vi "Am_Init.vi"(0 "COMPORT":refnum<visa-resource-name>="COM4", 1 "file path (dialog if empty)":path=path "C:/TetraLabGUI/Am_Init.py", 11 "error in (no error)":errorcluster, 13 "Open/Close Serial":bool) -> (3 "All Success":bool=TRUE, 4 "comport":refnum<visa-resource-name>="COM4", 15 "error out":errorcluster)   [LabVIEW 2018]
uses:
  <vilib>/Utility/error.llb/whitespace.ctl
  <vilib>/Utility/file.llb/Read Delimited Spreadsheet (string).vi
panel:
  in  "Run TetraSerial(t)":bool=TRUE
  out "size(s)":i32=17
  out "spreadsheet string":string="wr reg 0x02 0x0400;wr reg 0x03 0x0000;wr reg 0x04 1032;wr reg 0x05 4;wr reg 0x06 10;wr reg 0x08 256;wr reg 0x09 51;wr reg 0x0A 4;wr reg 0x0E 8000;wr reg 0x0F 0x5555;wr reg 0x10 0x0055;wr reg 0x11 0xAAAA;wr reg 0x12 0x00AA;wr reg 0x1A 0x0000;wr reg 0x1B 0x0000;wr reg 0x17 0x0300;wr reg 0x18 0x0000\r\n"
  out "Array":string[](array[string])=["wr reg 0x02 0x0400", "wr reg 0x03 0x0000", "wr reg 0x04 1032", "wr reg 0x05 4", "wr reg 0x06 10", "wr reg 0x08 256", "wr reg 0x09 51", "wr reg 0x0A 4", "wr reg 0x0E 8000", "wr reg 0x0F 0x5555", "wr reg 0x10 0x0055", "wr reg 0x11 0xAAAA", "wr reg 0x12 0x00AA", "wr reg 0x1A 0x0000", "wr reg 0x1B 0x0000", "wr reg 0x17 0x0300", "wr reg 0x18 0x0000"]
  out "Numeric":i32=18
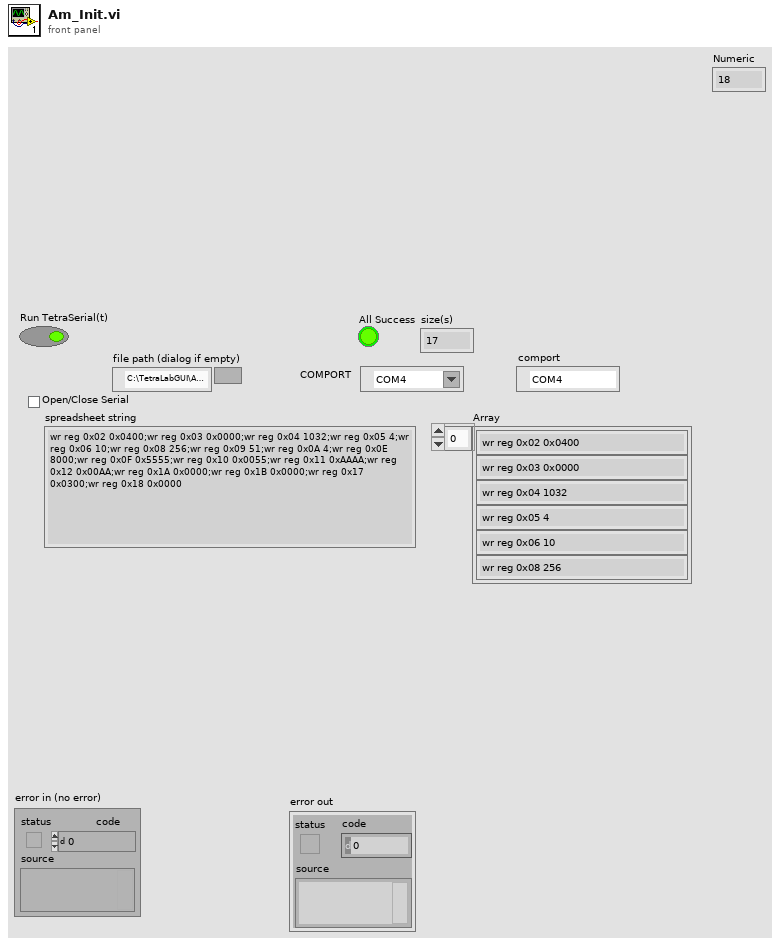
[diagram p1: front panel]
types:
  T1 = typedef "whitespace.ctl" = u16
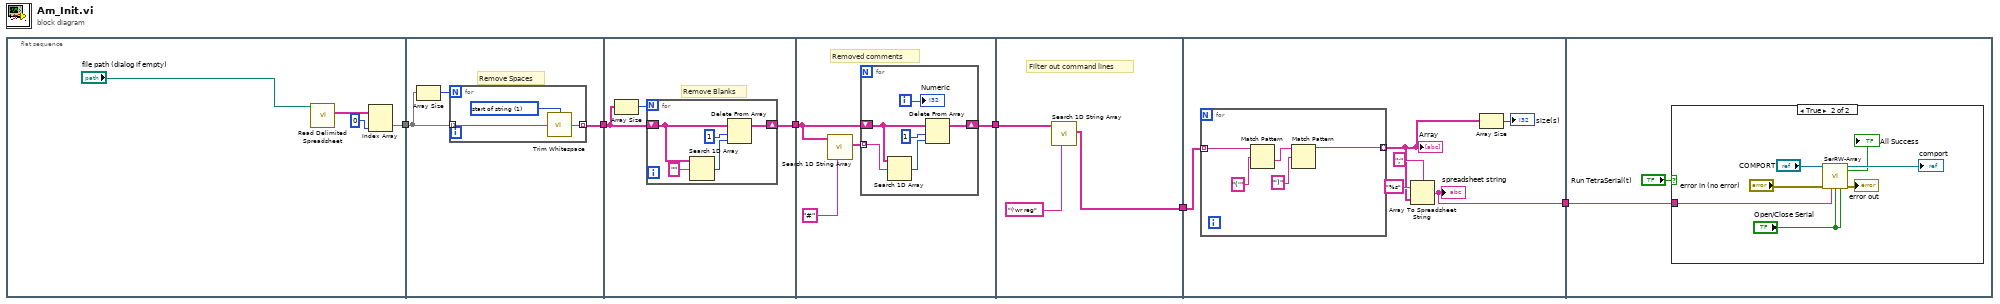
[diagram p0: block diagram]
diagram:
  n1 = flat-sequence {
    tunnel: [w7] -> w6
    tunnel: w6 -> [w12]
    tunnel: [w11] -> w5
    tunnel: w5 -> [w18]
    tunnel: [w17] -> w4
    tunnel: w4 -> [w25]
    tunnel: [w26] -> w3
    tunnel: w3 -> [w36]
    tunnel: [w35] -> w2
    tunnel: w2 -> [w43]
    tunnel: [w40] -> w1
    tunnel: w1 -> [w50]
    frame #0 {
      n2 = call-poly <vilib>:"Read Delimited Spreadsheet.vi"("file path (dialog if empty)"="file path (dialog if empty)") -> ("all rows"=w9:string[][])  [unwired: 9 in, 5 out]
      n3 = Index Array(array=w9, index (col)=0 ("disabled index (col)")) -> (element=w7:string[])  [unwired: 1 in]
    }
    frame #1 {
      # "Remove Spaces"
      n4 = Array Size(array=w12) -> (size(s)=w13:i32)
      n5 = for {
        N: w13 -> [_]
        tunnel: w12 -> [w16] mode=indexing
        tunnel: [w15] -> w11 mode=indexing
        w14 = T1 1 items=["both", "start of string", "end of string"] ("location (both)")
        n6 = call <vilib>:"Trim Whitespace.vi"("string"=w16, "location (both)"=w14) -> ("trimmed string"=w15:string)
      }
    }
    frame #2 {
      # "Remove Blanks"
      n7 = Array Size(array=w18) -> (size(s)=w19:i32)
      n8 = for {
        N: w19 -> [_]
        shift-right: [w21] -> w17
        shift-left: w18 -> [w24]
        n9 = Search 1D Array(1D array=w24, element="") -> (index of element=w23:i32)  [unwired: 1 in]
        n10 = Delete From Array(array=w24, length=1, index=w23) -> (array with subset deleted=w21:string[])  [unwired: 1 out]
      }
    }
    frame #3 {
      # "Removed comments"
      n11 = call "Search 1D String Array.vi"("Search Term"="#", "Input Array"=w25) -> ("Match Values"=w27:string[])  [unwired: 7 in, 2 out]
      n12 = for {
        shift-right: [w33] -> w26
        shift-left: w25 -> [w30]
        tunnel: w27 -> [w31] mode=indexing
        i -> [w32]
        n13 = Search 1D Array(1D array=w30, element=w31) -> (index of element=w29:i32)  [unwired: 1 in]
        n14 = Delete From Array(array=w30, length=1, index=w29) -> (array with subset deleted=w33:string[])  [unwired: 1 out]
        "Numeric" <- w32
      }
    }
    frame #4 {
      # "Filter out command lines"
      n15 = call "Search 1D String Array.vi"("Search Term"="('wr reg", "Input Array"=w36) -> ("Match Values"=w35:string[])  [unwired: 7 in, 2 out]
    }
    frame #5 {
      n16 = for {
        tunnel: w43 -> [w48] mode=indexing
        tunnel: [w44] -> w39 mode=indexing
        n17 = Match Pattern(string=w48, regular expression="('") -> (after substring=w46:string)  [unwired: 1 in, 3 out]
        n18 = Match Pattern(string=w46, regular expression="')") -> (before substring=w44:string)  [unwired: 1 in, 3 out]
      }
      "Array" <- w39
      n19 = Array To Spreadsheet String(delimiter (Tab)=";", array=w39, 3:"%s" ("format string")) -> (spreadsheet string=w40:string)
      "spreadsheet string" <- w40
      n20 = Array Size(array=w39) -> (size(s)=→"size(s)":i32)
    }
    frame #6 {
      n21 = case shown="True" "Run TetraSerial(t)" {
        tunnel: w50 -> [_ w55]
        frame False {
        }
        frame True {
          n22 = call "SerRW-Array.vi"("COMPORT"="COMPORT", "error in (no error)"="error in (no error)", "Command ( ; seperation)"=w55, "Open Serial"="Open/Close Serial", "Close Serial"="Open/Close Serial") -> ("All Success"=→"All Success":bool, "comport"=→"comport":refnum<visa-resource-name>, "error out"=→"error out":errorcluster)  [unwired: 4 in, 4 out]
        }
      }
    }
  }
